vi "actualizarIndicadores.vi"() -> ()   [LabVIEW 2026]
panel:
  in  "Enc_Cadera":refnum<vi>
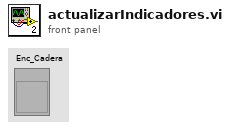
[diagram p1: front panel]
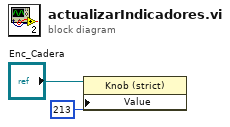
[diagram p0: block diagram]
diagram:
  n1 = property class="Knob (strict)"(reference="Enc_Cadera", "Value"=213) -> ()  [unwired: 1 in, 2 out]
